vi "DN4_BfdCntr_UDRead.vi"(8 "error in (no error)":errorcluster, 10 "stop?":bool, 11 "Task ID":u32) -> (0 "error out":errorcluster, 1 "stopped":bool, 2 "Array":i32[][](array[numeric]), 3 "Task out ID":u32)   [LabVIEW 2009]
uses:
  Windows/System32/AdvLvDaq.dll
panel:
  out "status":bool
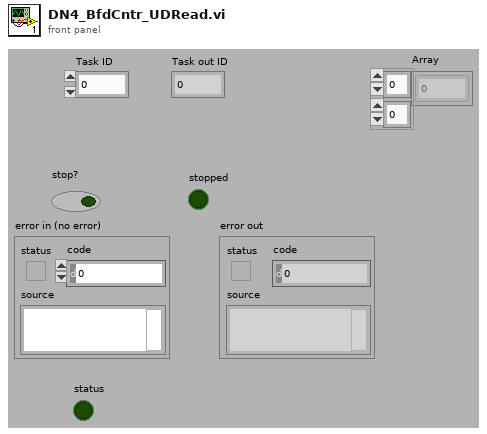
[diagram p1: front panel]
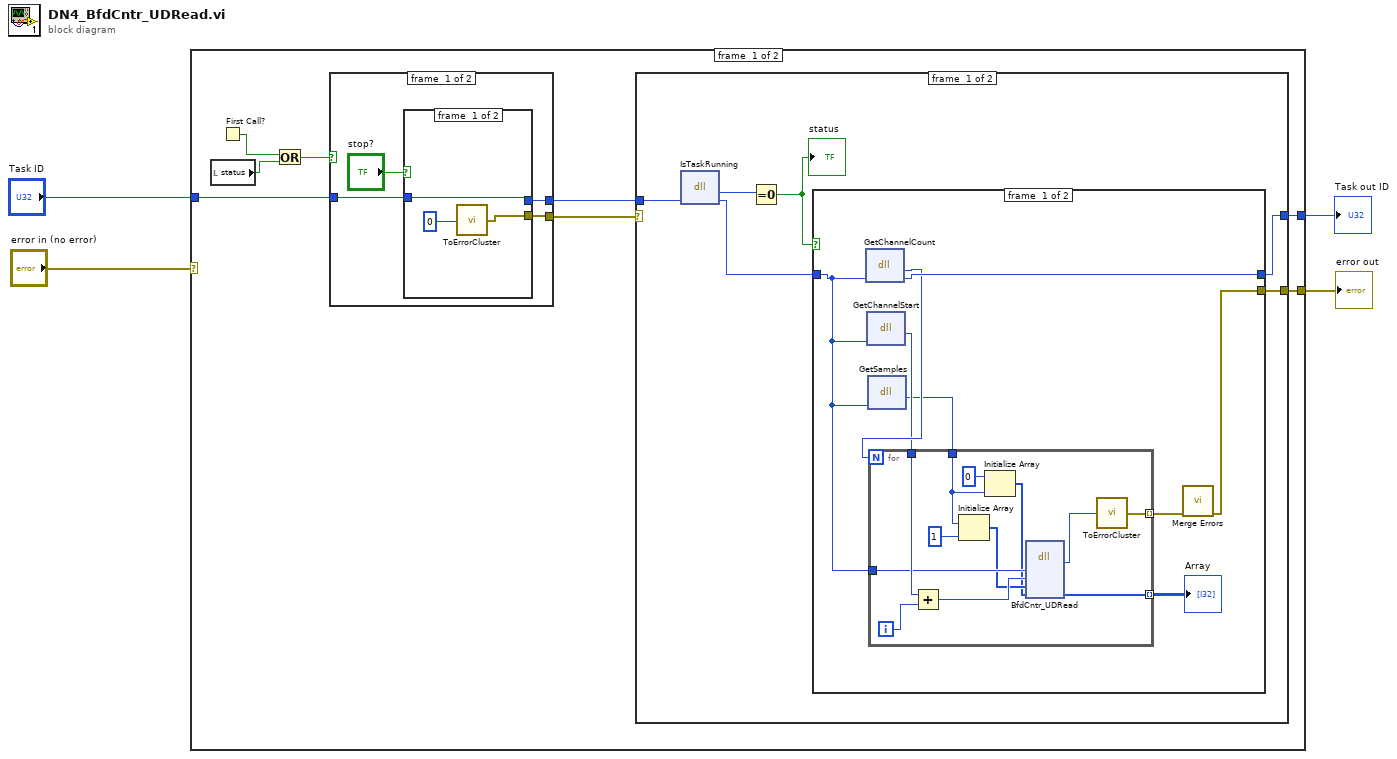
[diagram p0: block diagram]
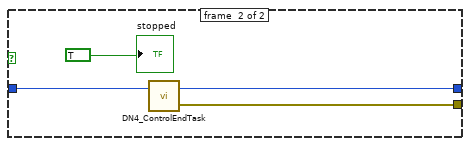
[diagram p2: hidden frame]
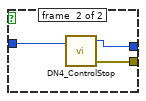
[diagram p4: hidden frame]
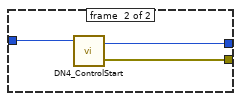
[diagram p5: hidden frame]
diagram:
  n1 = case shown="No Error" "error in (no error)" {
    selector: "error in (no error)" -> [_ w58]
    tunnel: "Task ID" -> [w9 w59]
    tunnel: [w7 w59] -> w2
    tunnel: [w6 w58] -> w1
    frame #0 {
      n2 = local read "status"() -> (w11:bool)
      n3 = First Call?() -> (First Call?: T/F=w12:bool)
      n4 = Or(x=w12, y=w11) -> (x .or. y?=w10:bool)
      n5 = case shown="True" w10 {
        tunnel: w9 -> [w47 w57]
        tunnel: [w46 w56] -> w8
        tunnel: [w45 w55] -> w5
        frame #0 {
          n6 = case shown="True" "stop?" {
            tunnel: w47 -> [w51 w54]
            tunnel: [w51 w53] -> w46
            tunnel: [w49 w52] -> w45
            frame #0 {
              n7 = call <userlib>:"ToErrorCluster.vi"("error code"=0) -> ("error out"=w49:errorcluster)
            }
            frame #1 {
              n8 = call <userlib>:"DN4_ControlStop.vi"("Task ID"=w54) -> ("error out"=w52:errorcluster, "Task ID"=w53:u32)  [unwired: 1 in, 2 out]
            }
          }
        }
        frame #1 {
          n9 = call <userlib>:"DN4_ControlStart.vi"("Task ID"=w57) -> ("error out"=w55:errorcluster, "Task ID"=w56:u32)  [unwired: 1 in, 1 out]
        }
      }
      n10 = case shown="No Error" w5 {
        selector: w5 -> [_ w43]
        tunnel: w8 -> [w18 w44]
        tunnel: [w14 w44] -> w7
        tunnel: [w13 w43] -> w6
        frame #0 {
          n11 = dll-call lib="C:/Windows/System32/AdvLvDaq.dll" fn="IsTaskRunning"("taskId"=w18) -> ("return type"=w17:i8, "taskId"=w15:u32)  [unwired: 3 in, 2 out]
          n12 = Equal To 0?(x=w17) -> (x = 0?=w16:bool)
          "status" <- w16
          n13 = case shown="True" w16 {
            tunnel: w15 -> [w23 w41]
            tunnel: [w26 w40] -> w14
            tunnel: [w19 w39] -> w13
            frame #0 {
              n14 = dll-call lib="C:/Windows/System32/AdvLvDaq.dll" fn="GetChannelCount"("taskId"=w23) -> ("return type"=w25:i32, "taskId"=w26:u32)  [unwired: 3 in, 2 out]
              n15 = dll-call lib="C:/Windows/System32/AdvLvDaq.dll" fn="GetChannelStart"("taskId"=w23) -> ("return type"=w24:i32)  [unwired: 4 in, 2 out]
              n16 = dll-call lib="C:/Windows/System32/AdvLvDaq.dll" fn="GetSamples"("taskId"=w23) -> ("return type"=w22:i32)  [unwired: 4 in, 2 out]
              n17 = for {
                N: w25 -> [_]
                tunnel: w24 -> [w37]
                tunnel: w23 -> [w35]
                tunnel: w22 -> [w33]
                tunnel: [w28] -> w20 mode=indexing
                tunnel: [w27] -> w21 mode=indexing
                i -> [w38]
                n18 = Add(x=w37, y=w38) -> (x+y=w36:i32)
                n19 = Initialize Array(w33, 1) -> (w34:i32[])
                n20 = Initialize Array(0, w33) -> (w30:i32[])
                n21 = dll-call lib="C:/Windows/System32/AdvLvDaq.dll" fn="BfdCntr_UDRead"("taskId"=w35, "cntr"=w36, "count"=w34, "data"=w30) -> ("return type"=w29:i32, "data"=w27:i32[])  [unwired: 5 in, 3 out]
                n22 = call <userlib>:"ToErrorCluster.vi"("error code"=w29) -> ("error out"=w28:errorcluster)
              }
              "Array" <- w21
              n23 = call <vilib>:"Merge Errors.vi"("error array in"=w20) -> ("error out"=w19:errorcluster)  [unwired: 3 in, 3 out]
            }
            frame #1 {
              n24 = call <userlib>:"DN4_ControlEndTask.vi"("Task ID"=w41) -> ("error out"=w39:errorcluster, "Task ID"=w40:u32)  [unwired: 1 in]
              "stopped" <- TRUE
            }
          }
        }
        frame #1 {
        }
      }
    }
    frame #1 {
    }
  }
  "Task out ID" <- w2
  "error out" <- w1
